vi "Q2.vi"() -> ()   [LabVIEW 2019]
uses:
  <vilib>/measure/NI_MABase.lvlib
  <vilib>/Analysis/NI_AAL_SigProc.lvlib
panel:
  in  "signal type":T1(ring)
  in  "frequency 2":dbl=10.0 format="%0.2p"
  in  "frequency":dbl=10.0 format="%0.2p"
  in  "m2":dbl
  in  "m1":dbl
  out "detected m2":dbl[](graph)
  out "fm2":waveform(dbl)(graph)
  out "fm1":waveform(dbl)(graph)
  out "detected m 1":dbl[](graph)
  in  "amplitude 4":dbl=1.0 format="%0.2p"
  in  "phase 4":dbl format="%.2p"
  in  "fc":cluster{"Fs":dbl, "#s":dbl}={"Fs"=1000.0, "#s"=1000.0} {"Fs" format="%.2p"}
  in  "amplitude 3":dbl=1.0 format="%0.2p"
  in  "phase 3":dbl format="%.2p"
  in  "amplitude 2":dbl=1.0 format="%0.2p"
  in  "phase 2":dbl format="%.2p"
  in  "fm 2":dbl=10.0 format="%0.2p"
  in  "amplitude":dbl=1.0 format="%0.2p"
  in  "phase":dbl format="%.2p"
  in  "fm1":dbl=10.0 format="%0.2p"
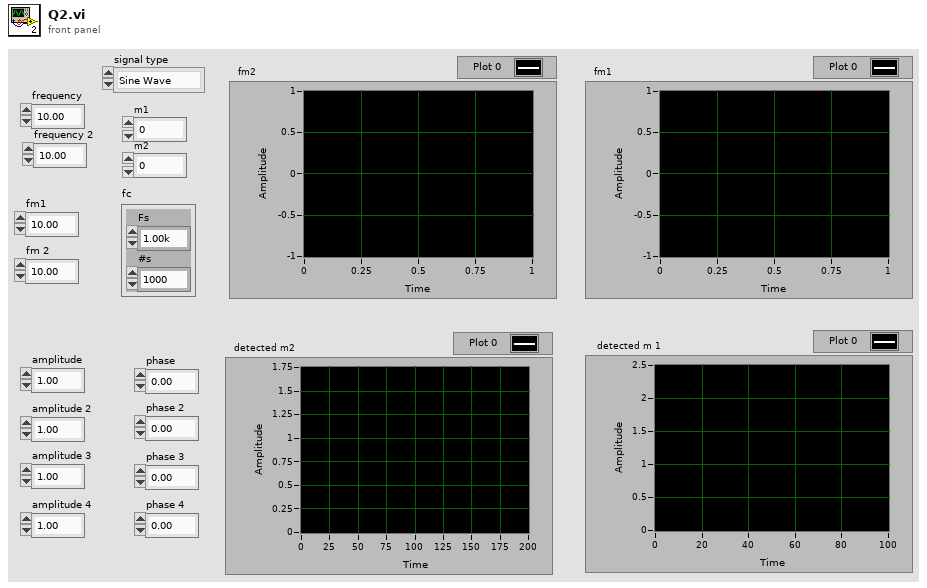
[diagram p1: front panel]
types:
  T1 = enum16{"Sine Wave", "Triangle Wave", "Square Wave", "Sawtooth Wave"}
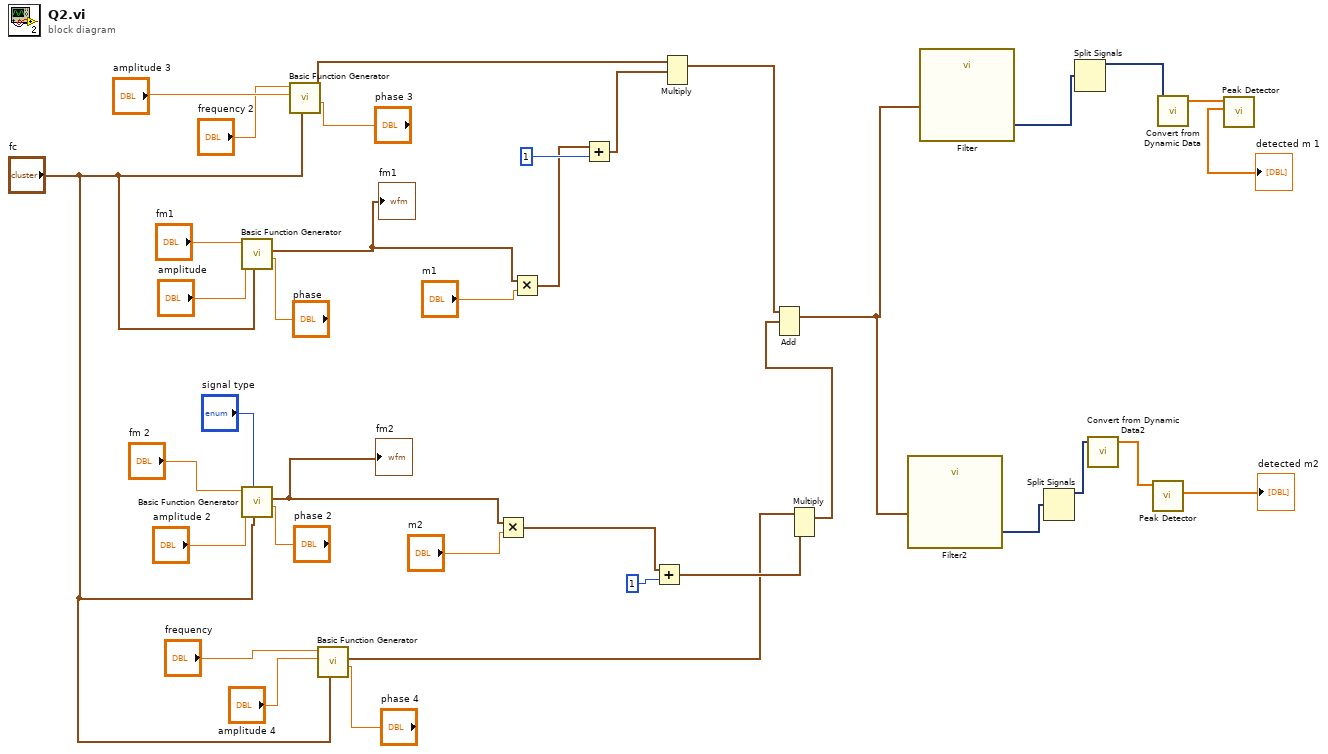
[diagram p0: block diagram]
diagram:
  n1 = call <vilib>:"Basic Function Generator.vi"("sampling info"="fc", "phase"="phase", "amplitude"="amplitude", "frequency"="fm1") -> ("signal out"=w13:waveform(dbl))  [unwired: 5 in, 2 out]
  "fm1" <- w13
  n2 = call <vilib>:"Basic Function Generator.vi"("sampling info"="fc", "signal type"="signal type", "phase"="phase 2", "amplitude"="amplitude 2", "frequency"="fm 2") -> ("signal out"=w10:waveform(dbl))  [unwired: 4 in, 2 out]
  "fm2" <- w10
  n3 = call <vilib>:"Basic Function Generator.vi"("sampling info"="fc", "phase"="phase 3", "amplitude"="amplitude 3", "frequency"="frequency 2") -> ("signal out"=w6:waveform(dbl))  [unwired: 5 in, 2 out]
  n4 = call <vilib>:"Basic Function Generator.vi"("sampling info"="fc", "phase"="phase 4", "amplitude"="amplitude 4", "frequency"="frequency") -> ("signal out"=w26:waveform(dbl))  [unwired: 5 in, 2 out]
  n5 = Multiply(x=w10, y="m2") -> (x*y=w9:waveform(dbl))
  n6 = Multiply(x=w13, y="m1") -> (x*y=w12:waveform(dbl))
  n7 = Add(x=w12, y=1) -> (x+y=w5:waveform(dbl))
  n8 = Add(x=w9, y=1) -> (x+y=w27:waveform(dbl))
  n9 = Multiply(1:w5, 2:w6) -> (0:w25:waveform(dbl))  [unwired: 1 in, 1 out]
  n10 = Multiply(1:w27, 2:w26) -> (0:w24:waveform(dbl))  [unwired: 1 in, 1 out]
  n11 = Add(1:w24, 2:w25) -> (0:w23:waveform(dbl))  [unwired: 1 in, 1 out]
  n12 = call "Filter2"("Signal"=w23) -> ("Filtered Signal"=w21:dynamicdata)  [unwired: 9 in, 1 out]
  n13 = call "Filter"("Signal"=w23) -> ("Filtered Signal"=w22:dynamicdata)  [unwired: 9 in, 1 out]
  n14 = Split Signals(w21) -> (w18:dynamicdata)  [unwired: 4 in, 3 out]
  n15 = Split Signals(w22) -> (w20:dynamicdata)  [unwired: 4 in, 3 out]
  n16 = call "Convert from Dynamic Data2"("Dynamic Data Type"=w18) -> ("Array"=w17:dbl[])  [unwired: 3 in]
  n17 = call <vilib>:"Peak Detector.vi"("X"=w17) -> ("Amplitudes"=→"detected m2":dbl[])  [unwired: 6 in, 4 out]
  n18 = call "Convert from Dynamic Data"("Dynamic Data Type"=w20) -> ("Array"=w19:dbl[])  [unwired: 3 in]
  n19 = call <vilib>:"Peak Detector.vi"("X"=w19) -> ("Amplitudes"=→"detected m 1":dbl[])  [unwired: 6 in, 4 out]
